vi "R45_1-RT.vi"() -> ()   [LabVIEW 2016]
uses:
  <vilib>/rvi/interface/nirviOpenFPGA/nirviOpenFPGA.xnode
  <vilib>/rvi/interface/nirviReadWriteControl/nirviReadWriteControl.xnode
  Slow-Switching-Control/FPGA Bitfiles/Controlsoftware2_FPGATarget10_R45-1-FPGA_wr0+Htmk8zo.lvbitx
  R45_1-FPGA.vi
  <vilib>/rvi/errors/niLvFpgaAdjustHostInterfaceError.vi
  <vilib>/Utility/error.llb/Error Cluster From Error Code.vi
  Gate Valve Readback.ctl
  Faraday Cup Readback.ctl
  Aperture Readback.ctl
  NiFpgaLv.dll
  <vilib>/Platform/TimedLoop/XDataNode/XDataNode.xnode
  <vilib>/Platform/TimedLoop/XDataNode/nitl_modes.ctl
  <vilib>/Platform/TimedLoop/XDataNode/XDNodeRunTimeDep.lvlib
  <vilib>/Platform/TimedLoop/XDataNode/wakeup.ctl
  <vilib>/Platform/TimedLoop/XDataNode/timing_clust.ctl
  Glassman Control.ctl
  <vilib>/FPGAPlugInAG/cRIO-9067/niLvFpga_Open_cRIO-9067.vi
  GV states.ctl
  Faraday cup states.ctl
  Aperture states.ctl
  GP307 cluster.ctl
panel:
  out "HV control loop error":errorcluster
  out "HV readback loop error":errorcluster
  out "Vac cluster loop error":errorcluster
  out "Cryo loop error":errorcluster
  out "Vac Cluster 1 Convectron 2":u8[](array[numeric])
  out "Vac Cluster 1 Ion Gauge 2":u8[](array[numeric])
  out "Switch Image Ion Gauge 1":dbl
  out "Switch Image Vac Cluster":T1
  out "Switch Image Convectron 1":dbl
  out "Vac Cluster 1 Convectron 1":u8[](array[numeric])
  out "Vac Cluster 1 Ion Gauge 1":u8[](array[numeric])
  out "Down-Steerer Voltage Set":dbl
  out "Down-Steerer HV Enable":bool
  out "Up-Steerer HV Enable":bool
  out "Up-Steerer Voltage Set":dbl
  out "Right-Steerer voltage set":dbl
  out "Right-Steerer HV Enable":bool
  out "Left-Steerer HV Enable":bool
  out "Left-Steerer voltage set":dbl
  out "Right Steerer readback.V-monitor":fxp<+/-,26,7>
  out "Right Steerer readback.I-monitor":fxp<+/-,26,5>
  out "Left Steerer readback.V-monitor":fxp<+/-,26,7>
  out "Left Steerer readback.I-monitor":fxp<+/-,26,5>
  out "Down Steerer readback.V-monitor":fxp<+/-,26,7>
  out "Down Steerer readback.I-monitor":fxp<+/-,26,5>
  out "Up Steerer readback.V-monitor":fxp<+/-,26,7>
  out "Up Steerer readback.I-monitor":fxp<+/-,26,5>
  out "Cryo 1st stage temp":u8[](array[numeric])
  out "Cryo On-time":u8[](array[numeric])
  out "Cryo status":u8[](array[numeric])
  out "Error Reporter":errorcluster
  out "Actuator-Sensor Loop error":errorcluster
  out "Interlock loop error":errorcluster
  out "Vac cluster 2 Ion Gauge Interlock":bool
  out "FC Status":T2
  out "Aperture Status":T3
  out "Switch Image Aperture Position":cluster{"IN sensor":bool, "OUT sensor":bool}
  out "Switch Image FC Position":cluster{"IN sensor":bool, "OUT sensor":bool}
  out "Beamline GV 1 status":T4
  out "Beamline GV 1 status":T5
  out "Cryo Pump GV status":T4
  out "Cryo Pump GV status":T5
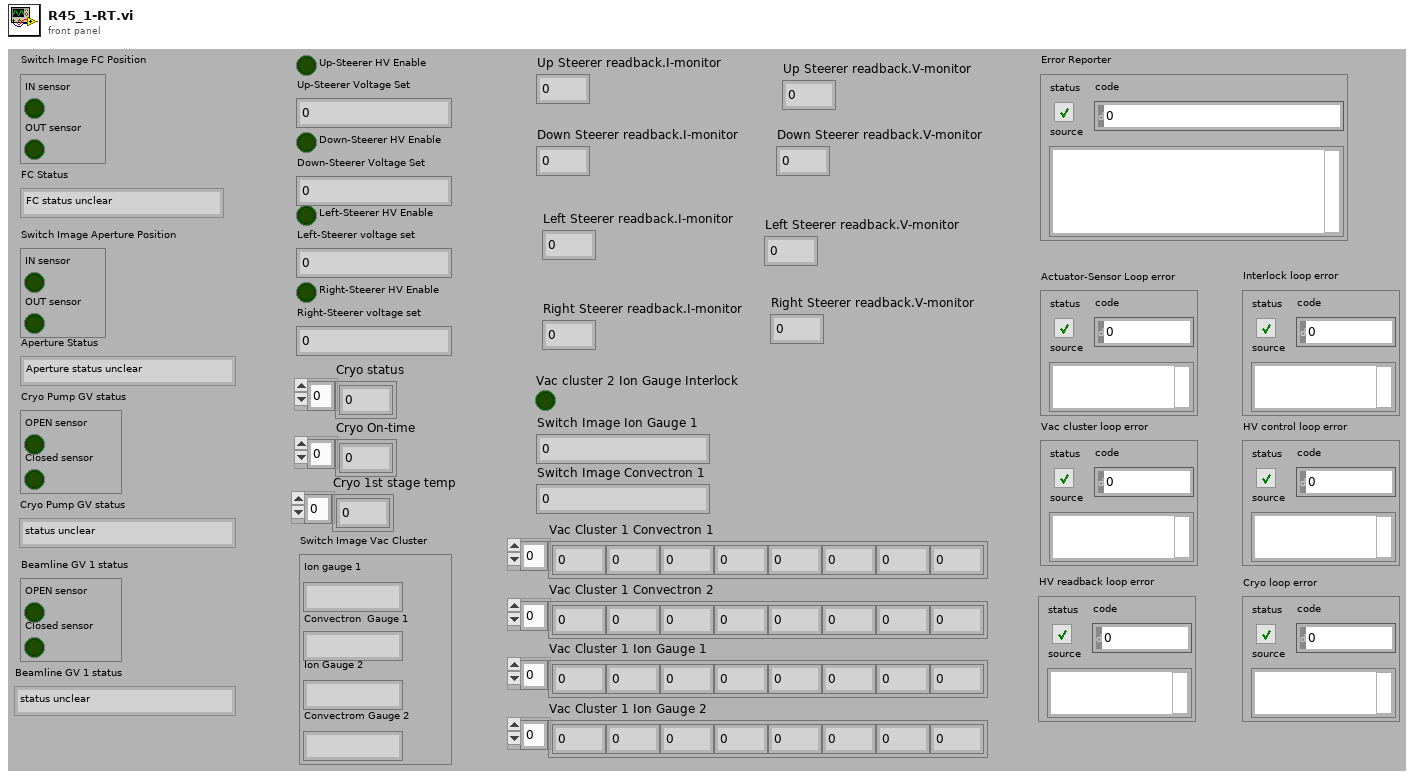
[diagram p1: front panel]
types:
  T1 = typedef "GP307 cluster.ctl" = cluster{"Ion gauge 1":string, "Convectron  Gauge 1 ":string, "Ion Gauge 2":string, "Convectrom Gauge 2":string}
  T2 = typedef "Faraday cup states.ctl" = enum16{"FC status unclear", "FC in", "FC out"}
  T3 = typedef "Aperture states.ctl" = enum16{"Aperture status unclear", "Aperture in", "Aperture out"}
  T4 = typedef "GV states.ctl" = enum16{"status unclear", "closed", "open"}
  T5 = cluster{"OPEN sensor":bool, "Closed sensor":bool}
  T6 = typedef "XDNodeRunTimeDep.lvlib/timing_clust.ctl" = cluster{"Expected End [f-1]":u64, "Actual End [f-1]":u64, "Finished Late? [f-1]":bool, "Expected End [i-1]":u64, "Actual End [i-1]":u64, "Finished Late? [i-1]":bool, "Expected Start [i]":u64, "Actual Start [i]":u64, "Expected Start [f]":u64, "Actual Start [f]":u64, "Source Name":string, "Structure Name":string, "Period":i64, "Deadline":i64, "Offset":i64, "Start":i64, "Priority":i32, "Timeout":i32, "Mode":T7, "Wakeup Reason":T8, "Error":errorcluster, "Source Type":string, "Secondary Source Type":string, "Global End Time":u64, "Global Start Time":u64, "Frame Duration":u64, "Iteration Duration":u64, "Assigned CPU":i32, "I/O Scan Engine Mode":u32}
  T7 = typedef "XDNodeRunTimeDep.lvlib/nitl_modes.ctl" = enum32{"No Change", "Process missed periods, maintain original phase", "Discard missed periods, maintain original phase", "Process missed periods, ignore original phase", "Discard missed periods, ignore original phase"}
  T8 = typedef "XDNodeRunTimeDep.lvlib/wakeup.ctl" = enum32{"Normal", "Aborted", "Asynchronous wakeup", "Timing source error", "Timed loop error", "Timeout"}
  T9 = typedef "Gate Valve Readback.ctl" = cluster{"OPEN sensor":bool, "Closed sensor":bool}
  T10 = typedef "Faraday Cup Readback.ctl" = cluster{"IN sensor":bool, "OUT sensor":bool}
  T11 = typedef "Aperture Readback.ctl" = cluster{"IN sensor":bool, "OUT sensor":bool}
  T12 = typedef "Glassman Control.ctl" = cluster{"V-program":fxp<+/-,20,7>, "HV Enable":bool}
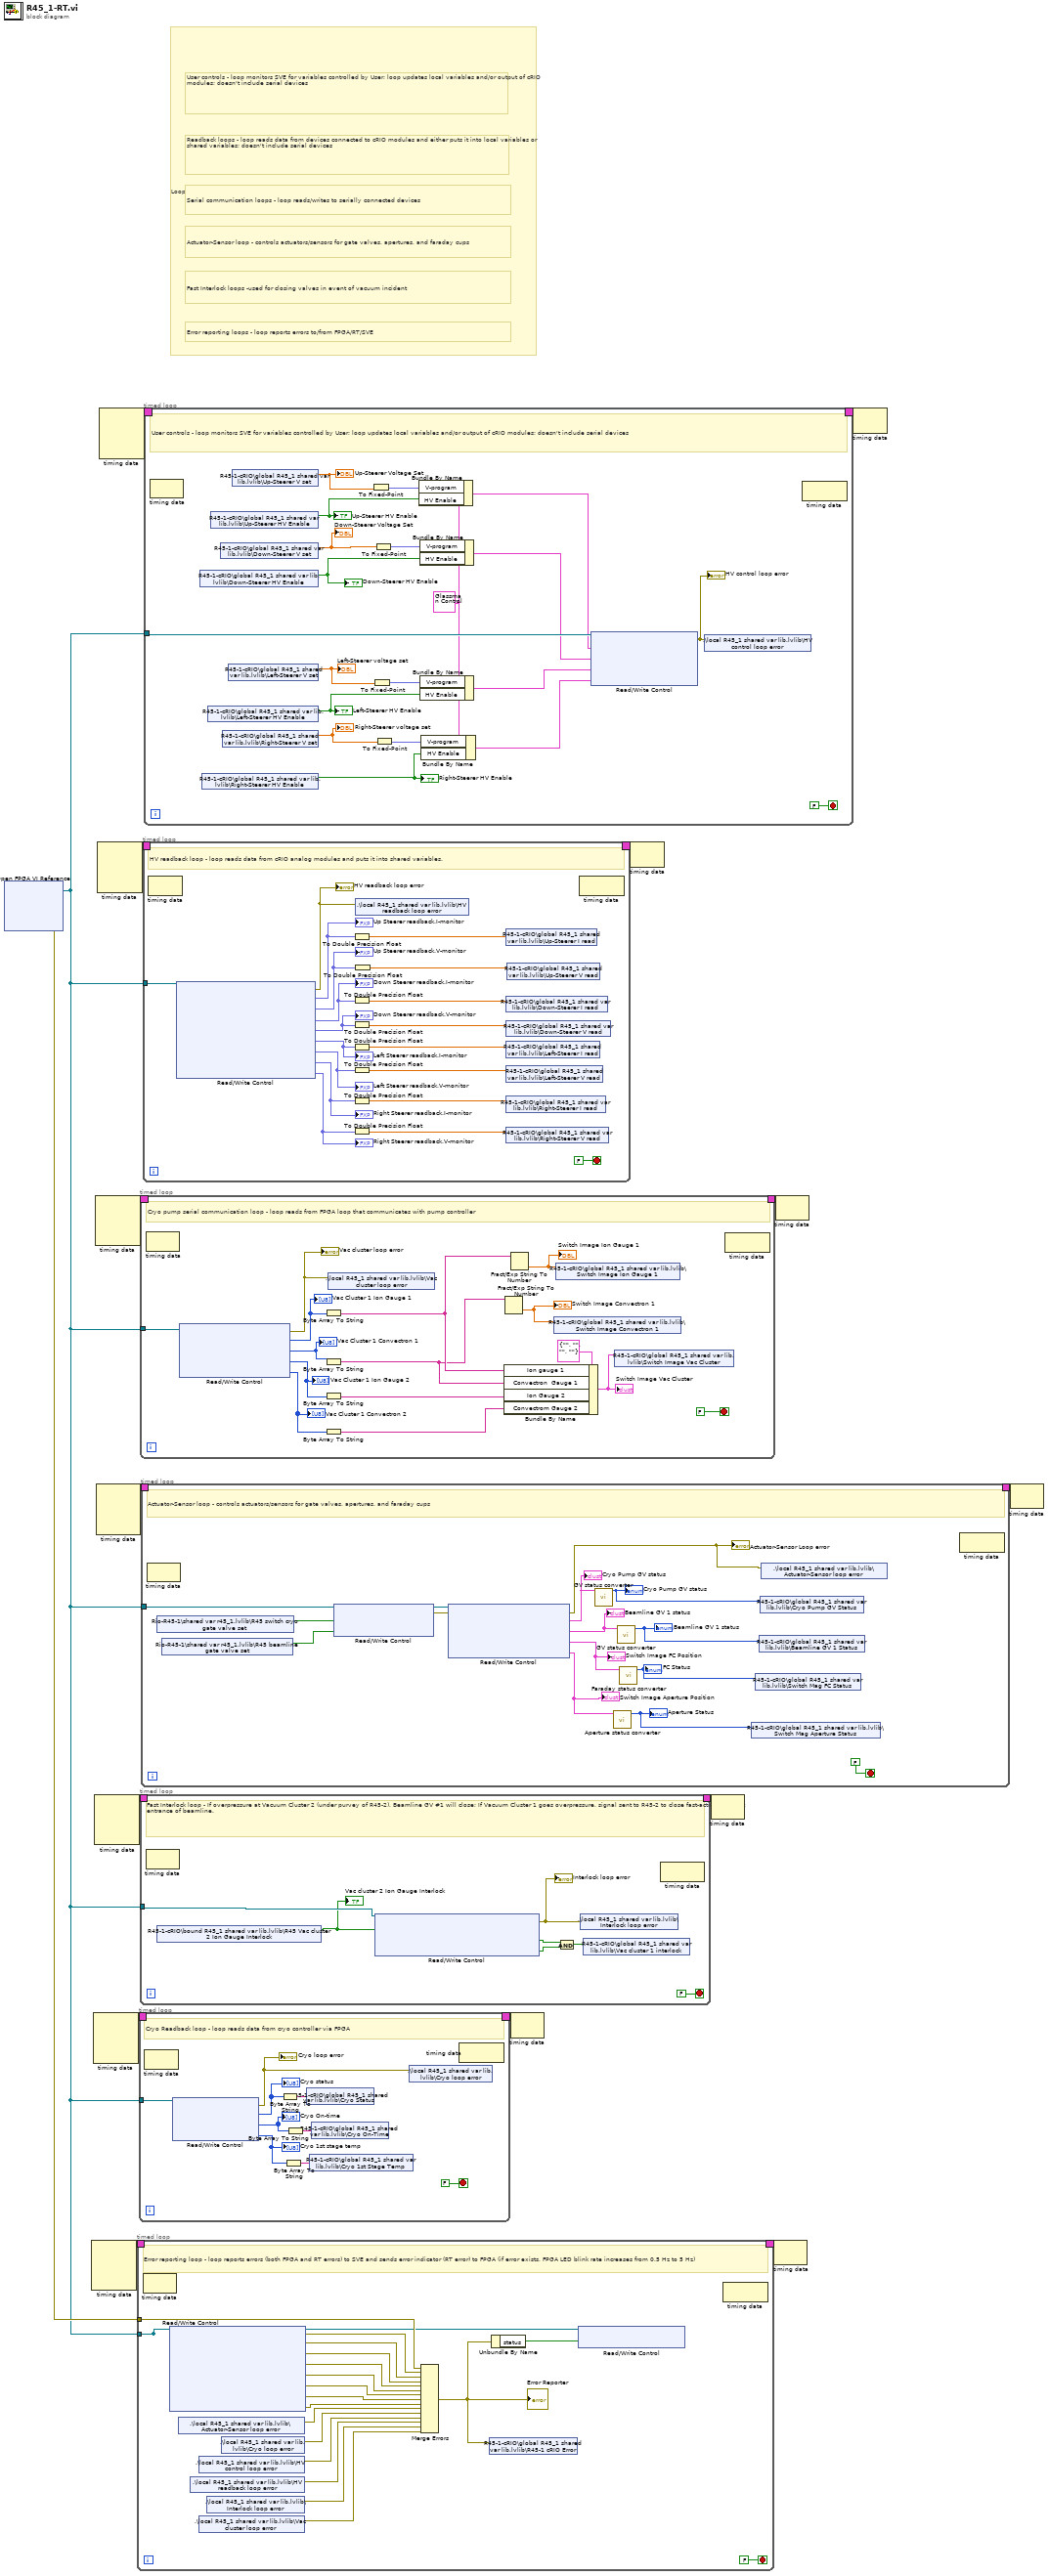
[diagram p0: block diagram]
diagram:
  # "Actuator-Sensor loop - controls actuators/sensors for gate valves, apertures, and faraday cups"
  # "Fast Interlock loops -used for closing valves in event of vacuum incident"
  # "Error reporting loops - loop reports errors to/from FPGA/RT/SVE"
  # "Serial communication loops - loop reads/writes to serially connected devices"
  # "Readback loops - loop reads data from devices connected to cRIO modules and either puts it into local variables or shared variables; doesn't include serial devices"
  # "User controls - loop monitors SVE for variables controlled by User; loop updates local variables and/or output of cRIO modules; doesn't include serial devices"
  # "Loop legend - loops are color coded by responsibility"
  n1 = xnode "Open FPGA VI Reference"() -> ("FPGA VI Reference Out"=w1:refnum<k20>, "error out"=w4:errorcluster)  [unwired: 2 in]
  n2 = node-c288() -> (w6:T6)  [unwired: 4 in]
  n3 = node-c288() -> (w3:T6)  [unwired: 4 in]
  n4 = node-c288() -> (w10:T6)  [unwired: 4 in]
  n5 = node-c288() -> (w14:T6)  [unwired: 4 in]
  n6 = node-c288() -> (w16:T6)  [unwired: 4 in]
  n7 = node-c288() -> (w8:T6)  [unwired: 4 in]
  n8 = node-c288() -> (w12:T6)  [unwired: 4 in]
  n9 = timed-loop {
    timing: w6 -> [_]
    timing-out: [_] -> w5
    tunnel: [w36] -> _
    tunnel: w1 -> [w36]
    tunnel: w4 -> [w35]
    stop <- FALSE stop-if-true
    # "Error reporting loop - loop reports errors (both FPGA and RT errors) to SVE and sends error indicator (RT error) to FPGA (if error exists, FPGA LED blink rate increases from 0.5 Hz to 5 Hz)"
    n10 = node-c288() -> ()  [unwired: 1 in, 1 out]
    n11 = xnode "Read/Write Control"("FPGA VI Reference In"=w36) -> ("FPGA VI Reference Out"=w19:refnum<k20>, "error out"=w34:errorcluster, "Vac and GV interlock error"=w33:errorcluster, "Position-Sensor readback error"=w32:errorcluster, "Cup-Aperture Control Loop Error"=w31:errorcluster, "Cryo pump error"=w30:errorcluster, "HV readback error"=w29:errorcluster, "HV Control error"=w28:errorcluster, "Vacuum Gauge 1 error"=w27:errorcluster)  [unwired: 1 in]
    n12 = shared-variable ".\\local R45_1 shared var lib.lvlib\\Actuator-Sensor loop error"() -> (w26:errorcluster)  [unwired: 1 in, 1 out]
    n13 = shared-variable ".\\local R45_1 shared var lib.lvlib\\HV readback loop error"() -> (w23:errorcluster)  [unwired: 1 in, 1 out]
    n14 = shared-variable ".\\local R45_1 shared var lib.lvlib\\HV control loop error"() -> (w24:errorcluster)  [unwired: 1 in, 1 out]
    n15 = shared-variable ".\\local R45_1 shared var lib.lvlib\\Vac cluster loop error"() -> (w21:errorcluster)  [unwired: 1 in, 1 out]
    n16 = shared-variable ".\\local R45_1 shared var lib.lvlib\\Interlock loop error"() -> (w22:errorcluster)  [unwired: 1 in, 1 out]
    n17 = shared-variable ".\\local R45_1 shared var lib.lvlib\\Cryo loop error"() -> (w25:errorcluster)  [unwired: 1 in, 1 out]
    n18 = Merge Errors(w35, w34, w33, w32, w31, w30, w29, w28, w27, w26, w25, w24, w23, w22, w21) -> (w20:errorcluster)
    "Error Reporter" <- w20
    n19 = shared-variable "R45-1-cRIO\\global R45_1 shared var lib.lvlib\\R45-1 cRIO Error"(w20) -> ()  [unwired: 1 in, 1 out]
    n20 = Unbundle By Name(w20) -> ("status"=w18:bool)
    n21 = xnode "Read/Write Control"("FPGA VI Reference In"=w19, "RT error"=w18) -> ()  [unwired: 1 in, 2 out]
    n22 = node-c288() -> ()  [unwired: 1 in, 1 out]
  }
  n23 = timed-loop {
    timing: w3 -> [_]
    timing-out: [_] -> w2
    tunnel: w1 -> [w46]
    stop <- FALSE stop-if-true
    # "Cryo Readback loop - loop reads data from cryo controller via FPGA"
    n24 = node-c288() -> ()  [unwired: 1 in, 1 out]
    n25 = xnode "Read/Write Control"("FPGA VI Reference In"=w46) -> ("error out"=w39:errorcluster, "Cryo status"=w43:u8[], "Cryo On-time"=w44:u8[], "Cryo 1st stage temp"=w45:u8[])  [unwired: 1 in, 1 out]
    "Cryo status" <- w43
    "Cryo On-time" <- w44
    "Cryo 1st stage temp" <- w45
    "Cryo loop error" <- w39
    n26 = Byte Array To String(unsigned byte array=w43) -> (string=w42:string)
    n27 = Byte Array To String(unsigned byte array=w45) -> (string=w40:string)
    n28 = Byte Array To String(unsigned byte array=w44) -> (string=w41:string)
    n29 = shared-variable "R45-1-cRIO\\global R45_1 shared var lib.lvlib\\Cryo Status"(w42) -> ()  [unwired: 1 in, 1 out]
    n30 = shared-variable "R45-1-cRIO\\global R45_1 shared var lib.lvlib\\Cryo 1st Stage Temp"(w40) -> ()  [unwired: 1 in, 1 out]
    n31 = shared-variable "R45-1-cRIO\\global R45_1 shared var lib.lvlib\\Cryo On-Time"(w41) -> ()  [unwired: 1 in, 1 out]
    n32 = shared-variable ".\\local R45_1 shared var lib.lvlib\\Cryo loop error"(w39) -> ()  [unwired: 1 in, 1 out]
    n33 = node-c288() -> ()  [unwired: 1 in, 1 out]
  }
  n34 = timed-loop {
    timing: w10 -> [_]
    timing-out: [_] -> w9
    tunnel: w1 -> [w53]
    stop <- FALSE stop-if-true
    # "Fast Interlock loop - If overpressure at Vacuum Cluster 2 (under purvey of R45-2), Beamline GV #1 will close; If Vacuum Cluster 1 goes overpressure, signal sent to R45-2 to close fast-acting valve at entrance of beamline."
    n35 = node-c288() -> ()  [unwired: 1 in, 1 out]
    n36 = shared-variable "R45-1-cRIO\\bound R45_1 shared var lib.lvlib\\R45 Vac cluster 2 Ion Gauge Interlock"() -> (w52:bool)  [unwired: 1 in, 1 out]
    "Vac cluster 2 Ion Gauge Interlock" <- w52
    n37 = xnode "Read/Write Control"("FPGA VI Reference In"=w53, "Vac cluster 2 Ion Gauge Interlock"=w52) -> ("error out"=w51:errorcluster, "Vac cluster 1 Ion Guage Interlock"=w56:bool, "Vac cluster 1 Convectron Guage Interlock"=w55:bool)  [unwired: 1 in, 1 out]
    "Interlock loop error" <- w51
    n38 = And(x=w56, y=w55) -> (x .and. y?=w54:bool)
    n39 = shared-variable ".\\local R45_1 shared var lib.lvlib\\Interlock loop error"(w51) -> ()  [unwired: 1 in, 1 out]
    n40 = shared-variable "R45-1-cRIO\\global R45_1 shared var lib.lvlib\\Vac cluster 1 interlock"(w54) -> ()  [unwired: 1 in, 1 out]
    n41 = node-c288() -> ()  [unwired: 1 in, 1 out]
  }
  n42 = timed-loop {
    tunnel: w1 -> [w68]
    timing: w14 -> [_]
    timing-out: [_] -> w13
    stop <- FALSE stop-if-true
    # "Cryo pump serial communication loop - loop reads from FPGA loop that communicates with pump controller"
    n43 = node-c288() -> ()  [unwired: 1 in, 1 out]
    n44 = xnode "Read/Write Control"("FPGA VI Reference In"=w68) -> ("error out"=w61:errorcluster, "Vac Cluster 1 Ion Gauge 1"=w69:u8[], "Vac Cluster 1 Convectron 1"=w64:u8[], "Vac Cluster 1 Ion Gauge 2"=w70:u8[], "Vac Cluster 1 Convectron 2"=w71:u8[])  [unwired: 1 in, 1 out]
    "Vac Cluster 1 Ion Gauge 1" <- w69
    "Vac Cluster 1 Convectron 1" <- w64
    "Vac Cluster 1 Ion Gauge 2" <- w70
    "Vac Cluster 1 Convectron 2" <- w71
    "Vac cluster loop error" <- w61
    n45 = Byte Array To String(unsigned byte array=w69) -> (string=w65:string)
    n46 = Byte Array To String(unsigned byte array=w64) -> (string=w63:string)
    n47 = Byte Array To String(unsigned byte array=w70) -> (string=w72:string)
    n48 = Byte Array To String(unsigned byte array=w71) -> (string=w73:string)
    n49 = shared-variable ".\\local R45_1 shared var lib.lvlib\\Vac cluster loop error"(w61) -> ()  [unwired: 1 in, 1 out]
    n50 = Bundle By Name(cluster=T1 {"Ion gauge 1"="", "Convectron  Gauge 1 "="", "Ion Gauge 2"="", "Convectrom Gauge 2"=""} ("Ion gauge cluster control"), "Ion gauge 1"=w65, "Convectron  Gauge 1"=w63, "Ion Gauge 2"=w72, "Convectrom Gauge 2"=w73) -> (w66:T1)
    "Switch Image Vac Cluster" <- w66
    n51 = Fract/Exp String To Number(string=w63) -> (number=w60:dbl)  [unwired: 3 in, 1 out]
    "Switch Image Convectron 1" <- w60
    n52 = Fract/Exp String To Number(string=w65) -> (number=w62:dbl)  [unwired: 3 in, 1 out]
    "Switch Image Ion Gauge 1" <- w62
    n53 = shared-variable "R45-1-cRIO\\global R45_1 shared var lib.lvlib\\Switch Image Convectron 1"(w60) -> ()  [unwired: 1 in, 1 out]
    n54 = shared-variable "R45-1-cRIO\\global R45_1 shared var lib.lvlib\\Switch Image Ion Gauge 1"(w62) -> ()  [unwired: 1 in, 1 out]
    n55 = shared-variable "R45-1-cRIO\\global R45_1 shared var lib.lvlib\\Switch Image Vac Cluster"(w66) -> ()  [unwired: 1 in, 1 out]
    n56 = node-c288() -> ()  [unwired: 1 in, 1 out]
  }
  n57 = timed-loop {
    tunnel: w1 -> [w89]
    timing: w16 -> [_]
    timing-out: [_] -> w15
    stop <- FALSE stop-if-true
    # "Actuator-Sensor loop - controls actuators/sensors for gate valves, apertures, and faraday cups"
    n58 = node-c288() -> ()  [unwired: 1 in, 1 out]
    n59 = shared-variable "Rio-R45-1\\shared var r45_1.lvlib\\R45 switch cryo gate valve set"() -> (w90:bool)  [unwired: 1 in, 1 out]
    n60 = shared-variable "Rio-R45-1\\shared var r45_1.lvlib\\R45 beamline gate valve set"() -> (w87:bool)  [unwired: 1 in, 1 out]
    n61 = xnode "Read/Write Control"("FPGA VI Reference In"=w89, "Cryo GV actuator"=w90, "Beamline GV 1 actuator"=w87) -> ("FPGA VI Reference Out"=w86:refnum<k20>, "error out"=w85:errorcluster)  [unwired: 1 in]
    n62 = xnode "Read/Write Control"("FPGA VI Reference In"=w86, "error in"=w85) -> ("error out"=w76:errorcluster, "Cryo Pump GV position"=w83:T9, "Beamline GV 1 position"=w81:T9, "Switch Mag FC Position"=w80:T10, "Switch Mag Aperture Position"=w79:T11)  [unwired: 1 out]
    "Cryo Pump GV status" <- w83
    "Beamline GV 1 status" <- w81
    "Switch Image FC Position" <- w80
    "Switch Image Aperture Position" <- w79
    "Actuator-Sensor Loop error" <- w76
    n63 = call "GV status converter.vi"("Gate Valve"=w83) -> ("GV Status"=w84:T4)  [unwired: 10 in]
    "Cryo Pump GV status" <- w84
    n64 = call "Aperture status converter.vi"("Aperture Position"=w79) -> ("Aperture Status"=w78:T3)  [unwired: 10 in]
    "Aperture Status" <- w78
    n65 = call "GV status converter.vi"("Gate Valve"=w81) -> ("GV Status"=w82:T4)  [unwired: 10 in]
    "Beamline GV 1 status" <- w82
    n66 = call "Faraday status converter.vi"("FC Position"=w80) -> ("FC Status"=w77:T2)  [unwired: 10 in]
    "FC Status" <- w77
    n67 = shared-variable "R45-1-cRIO\\global R45_1 shared var lib.lvlib\\Switch Mag Aperture Status"(w78) -> ()  [unwired: 1 in, 1 out]
    n68 = shared-variable "R45-1-cRIO\\global R45_1 shared var lib.lvlib\\Switch Mag FC Status"(w77) -> ()  [unwired: 1 in, 1 out]
    n69 = shared-variable "R45-1-cRIO\\global R45_1 shared var lib.lvlib\\Beamline GV 1 Status"(w82) -> ()  [unwired: 1 in, 1 out]
    n70 = shared-variable "R45-1-cRIO\\global R45_1 shared var lib.lvlib\\Cryo Pump GV Status"(w84) -> ()  [unwired: 1 in, 1 out]
    n71 = shared-variable ".\\local R45_1 shared var lib.lvlib\\Actuator-Sensor loop error"(w76) -> ()  [unwired: 1 in, 1 out]
    n72 = node-c288() -> ()  [unwired: 1 in, 1 out]
  }
  n73 = timed-loop {
    timing: w8 -> [_]
    timing-out: [_] -> w7
    tunnel: w1 -> [w111]
    stop <- FALSE stop-if-true
    # "HV readback loop - loop reads data from cRIO analog modules and puts it into shared variables."
    n74 = node-c288() -> ()  [unwired: 1 in, 1 out]
    n75 = xnode "Read/Write Control"("FPGA VI Reference In"=w111) -> ("error out"=w109:errorcluster, "Up Steerer readback.I-monitor"=w108:fxp<+/-,26,5>, "Up Steerer readback.V-monitor"=w107:fxp<+/-,26,7>, "Down Steerer readback.I-monitor"=w106:fxp<+/-,26,5>, "Down Steerer readback.V-monitor"=w105:fxp<+/-,26,7>, "Left Steerer readback.I-monitor"=w104:fxp<+/-,26,5>, "Left Steerer readback.V-monitor"=w103:fxp<+/-,26,7>, "Right Steerer readback.I-monitor"=w102:fxp<+/-,26,5>, "Right Steerer readback.V-monitor"=w101:fxp<+/-,26,7>)  [unwired: 1 in, 1 out]
    "Up Steerer readback.I-monitor" <- w108
    "Up Steerer readback.V-monitor" <- w107
    "Down Steerer readback.I-monitor" <- w106
    "Down Steerer readback.V-monitor" <- w105
    "Left Steerer readback.I-monitor" <- w104
    "Left Steerer readback.V-monitor" <- w103
    "Right Steerer readback.I-monitor" <- w102
    "Right Steerer readback.V-monitor" <- w101
    "HV readback loop error" <- w109
    n76 = To Double Precision Float(number=w108) -> (double precision float=w100:dbl)
    n77 = To Double Precision Float(number=w106) -> (double precision float=w97:dbl)
    n78 = To Double Precision Float(number=w105) -> (double precision float=w96:dbl)
    n79 = To Double Precision Float(number=w104) -> (double precision float=w95:dbl)
    n80 = To Double Precision Float(number=w103) -> (double precision float=w94:dbl)
    n81 = To Double Precision Float(number=w102) -> (double precision float=w93:dbl)
    n82 = To Double Precision Float(number=w101) -> (double precision float=w99:dbl)
    n83 = To Double Precision Float(number=w107) -> (double precision float=w98:dbl)
    n84 = shared-variable ".\\local R45_1 shared var lib.lvlib\\HV readback loop error"(w109) -> ()  [unwired: 1 in, 1 out]
    n85 = shared-variable "R45-1-cRIO\\global R45_1 shared var lib.lvlib\\Down-Steerer I read"(w97) -> ()  [unwired: 1 in, 1 out]
    n86 = shared-variable "R45-1-cRIO\\global R45_1 shared var lib.lvlib\\Up-Steerer I read"(w100) -> ()  [unwired: 1 in, 1 out]
    n87 = shared-variable "R45-1-cRIO\\global R45_1 shared var lib.lvlib\\Down-Steerer V read"(w96) -> ()  [unwired: 1 in, 1 out]
    n88 = shared-variable "R45-1-cRIO\\global R45_1 shared var lib.lvlib\\Left-Steerer I read"(w95) -> ()  [unwired: 1 in, 1 out]
    n89 = shared-variable "R45-1-cRIO\\global R45_1 shared var lib.lvlib\\Left-Steerer V read"(w94) -> ()  [unwired: 1 in, 1 out]
    n90 = shared-variable "R45-1-cRIO\\global R45_1 shared var lib.lvlib\\Right-Steerer I read"(w93) -> ()  [unwired: 1 in, 1 out]
    n91 = shared-variable "R45-1-cRIO\\global R45_1 shared var lib.lvlib\\Right-Steerer V read"(w99) -> ()  [unwired: 1 in, 1 out]
    n92 = shared-variable "R45-1-cRIO\\global R45_1 shared var lib.lvlib\\Up-Steerer V read"(w98) -> ()  [unwired: 1 in, 1 out]
    n93 = node-c288() -> ()  [unwired: 1 in, 1 out]
  }
  n94 = timed-loop {
    tunnel: w1 -> [w133]
    timing: w12 -> [_]
    timing-out: [_] -> w11
    stop <- FALSE stop-if-true
    w122 = T12 {"V-program"=0.0, "HV Enable"=FALSE} ("Glassman Control")
    # "User controls - loop monitors SVE for variables controlled by User; loop updates local variables and/or output of cRIO modules; doesn't include serial devices"
    n95 = node-c288() -> ()  [unwired: 1 in, 1 out]
    n96 = shared-variable "R45-1-cRIO\\global R45_1 shared var lib.lvlib\\Down-Steerer HV Enable"() -> (w118:bool)  [unwired: 1 in, 1 out]
    "Down-Steerer HV Enable" <- w118
    n97 = shared-variable "R45-1-cRIO\\global R45_1 shared var lib.lvlib\\Right-Steerer HV Enable"() -> (w114:bool)  [unwired: 1 in, 1 out]
    "Right-Steerer HV Enable" <- w114
    n98 = shared-variable "R45-1-cRIO\\global R45_1 shared var lib.lvlib\\Left-Steerer HV Enable"() -> (w116:bool)  [unwired: 1 in, 1 out]
    "Left-Steerer HV Enable" <- w116
    n99 = shared-variable "R45-1-cRIO\\global R45_1 shared var lib.lvlib\\Up-Steerer HV Enable"() -> (w121:bool)  [unwired: 1 in, 1 out]
    "Up-Steerer HV Enable" <- w121
    n100 = shared-variable "R45-1-cRIO\\global R45_1 shared var lib.lvlib\\Down-Steerer V set"() -> (w119:dbl)  [unwired: 1 in, 1 out]
    "Down-Steerer Voltage Set" <- w119
    n101 = shared-variable "R45-1-cRIO\\global R45_1 shared var lib.lvlib\\Right-Steerer V set"() -> (w115:dbl)  [unwired: 1 in, 1 out]
    "Right-Steerer voltage set" <- w115
    n102 = shared-variable "R45-1-cRIO\\global R45_1 shared var lib.lvlib\\Left-Steerer V set"() -> (w117:dbl)  [unwired: 1 in, 1 out]
    "Left-Steerer voltage set" <- w117
    n103 = shared-variable "R45-1-cRIO\\global R45_1 shared var lib.lvlib\\Up-Steerer V set"() -> (w120:dbl)  [unwired: 1 in, 1 out]
    "Up-Steerer Voltage Set" <- w120
    n104 = To Fixed-Point(number=w120) -> (fixed-point=w126:fxp<+/-,20,5>)  [unwired: 1 in]
    n105 = To Fixed-Point(number=w117) -> (fixed-point=w130:fxp<+/-,20,5>)  [unwired: 1 in]
    n106 = To Fixed-Point(number=w119) -> (fixed-point=w125:fxp<+/-,20,5>)  [unwired: 1 in]
    n107 = To Fixed-Point(number=w115) -> (fixed-point=w129:fxp<+/-,20,5>)  [unwired: 1 in]
    n108 = Bundle By Name(cluster=w122, "V-program"=w126, "HV Enable"=w121) -> (w123:T12)
    n109 = Bundle By Name(cluster=w122, "V-program"=w125, "HV Enable"=w118) -> (w124:T12)
    n110 = Bundle By Name(cluster=w122, "V-program"=w130, "HV Enable"=w116) -> (w127:T12)
    n111 = Bundle By Name(cluster=w122, "V-program"=w129, "HV Enable"=w114) -> (w128:T12)
    n112 = xnode "Read/Write Control"("FPGA VI Reference In"=w133, "Up Steerer Voltage set"=w123, "Down Steerer Voltage set"=w124, "Left Steerer Voltage set"=w127, "Right Steerer Voltage set"=w128) -> ("error out"=w131:errorcluster)  [unwired: 1 in, 1 out]
    "HV control loop error" <- w131
    n113 = shared-variable ".\\local R45_1 shared var lib.lvlib\\HV control loop error"(w131) -> ()  [unwired: 1 in, 1 out]
    n114 = node-c288() -> ()  [unwired: 1 in, 1 out]
  }
  n115 = node-c288(w2) -> ()  [unwired: 1 out]
  n116 = node-c288(w7) -> ()  [unwired: 1 out]
  n117 = node-c288(w9) -> ()  [unwired: 1 out]
  n118 = node-c288(w5) -> ()  [unwired: 1 out]
  n119 = node-c288(w13) -> ()  [unwired: 1 out]
  n120 = node-c288(w11) -> ()  [unwired: 1 out]
  n121 = node-c288(w15) -> ()  [unwired: 1 out]
